vi "Set Window Title.vi"(8 "error in (no error)":errorcluster, 10 "FP Window:Title":string, 11 "Panel in":refnum<class "Panel.lvclass">) -> (0 "error out":errorcluster, 3 "Panel out":refnum<class "Panel.lvclass">)   [LabVIEW 2021, in "Panel.lvlib" / "Panel.lvclass"]
uses:
  Panel.lvclass
  Panel.lvclass/Panel.ctl
  Station/Station Actor/Station.lvclass
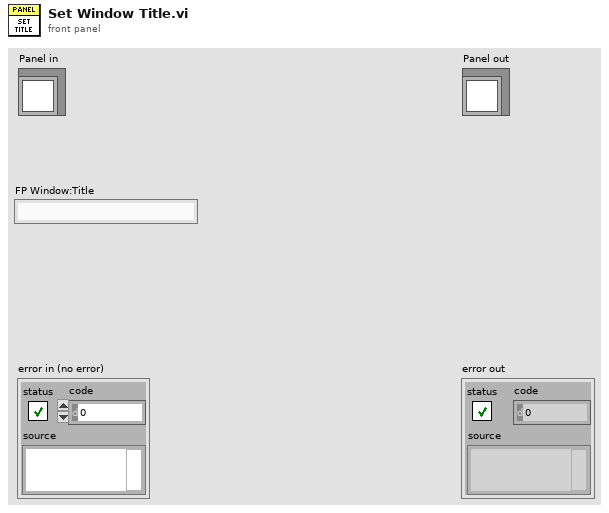
[diagram p1: front panel]
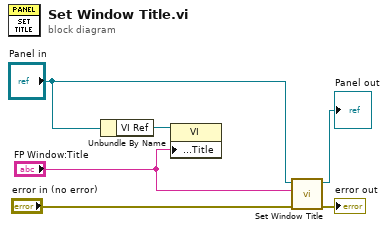
[diagram p0: block diagram]
diagram:
  n1 = Unbundle By Name("Panel in") -> ("VI Ref"=w4:refnum<vi>)
  n2 = property class="VI"(reference=w4, "Front Panel.Title"="FP Window:Title") -> ()  [unwired: 1 in, 2 out]
  n3 = call-parent "Set Window Title.vi"("error in (no error)"="error in (no error)", "FP Window:Title"="FP Window:Title", "Station in"="Panel in") -> ("error out"=→"error out":errorcluster, "Station out"=→"Panel out":refnum<class "Panel.lvclass">)  [unwired: 7 in]
